vi "stopSender.vi"(8 "error in (no error)":errorcluster, 11 "TcpServerBase in":refnum<class "TcpServerBase.lvclass">) -> (0 "error out":errorcluster, 3 "TcpServerBase out":refnum<class "TcpServerBase.lvclass">)   [LabVIEW 2018, in "TcpServerBase.lvclass"]
doc: "Send a signal to stop the Sender Loop (inside of readWritePacket.vi)"
uses:
  TcpServerBase.lvclass
  typedef/tcpPacketTypeDef.ctl
  TcpServerBase.lvclass/TcpServerBase.ctl
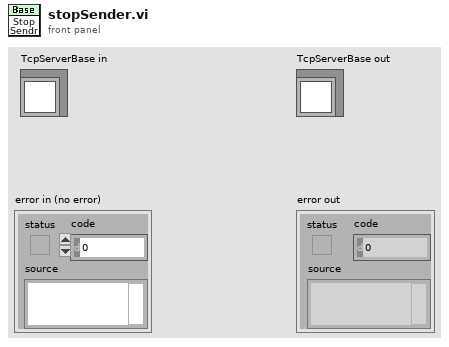
[diagram p1: front panel]
types:
  T1 = typedef "TcpServerBase.lvclass/tcpPacketTypeDef.ctl" = cluster{"packet":string, "firstPacket":bool, "firstConnection":bool}
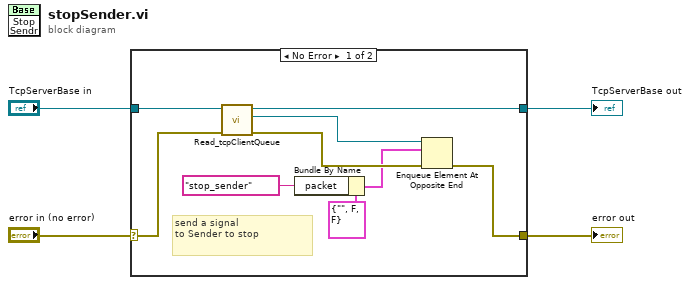
[diagram p0: block diagram]
diagram:
  n1 = case shown="No Error" "error in (no error)" {
    selector: "error in (no error)" -> [w9 w15]
    tunnel: [w8 w15] -> w3
    tunnel: [w11 w14] -> w1
    tunnel: "TcpServerBase in" -> [w12 w14]
    frame No Error {
      # "send a signal \nto Sender to stop"
      n2 = call "Read_tcpClientQueue.vi"("error in (no error)"=w9, "TcpServerBase in"=w12) -> ("error out"=w10:errorcluster, "tcpClientQueue"=w13:refnum<queue>, "TcpServerBase out"=w11:refnum<class "TcpServerBase.lvclass">)  [unwired: 7 in]
      n3 = Bundle By Name(cluster=T1 {"packet"="", "firstPacket"=FALSE, "firstConnection"=FALSE} ("packetConnID"), "packet"="stop_sender") -> (w5:T1)
      n4 = Enqueue Element At Opposite End(queue=w13, element=w5, error in (no error)=w10) -> (error out=w8:errorcluster)  [unwired: 1 in, 2 out]
    }
    frame Error {
    }
  }
  "error out" <- w3
  "TcpServerBase out" <- w1
